vi "WPI_GyroRomiGetAngle.vi"(8 "error in":T1, 11 "GyroDevRef":typedef) -> (0 "error out":T1, 1 "Anglular Rate":T2, 2 "Angle":T2, 3 "GyroDevRef":typedef, 4 "Calibrated?":boolean)   [LabVIEW 2019]
doc: "Returns the angle, in degrees from the original heading, that the robot is currently facing.\n\nThis software is licensed. Open the labview\\readme\\WPI Robotics Library Open Source License.txt file for more information."
uses:
  <vilib>/Rock Robotics/WPI/Gyro/WPI_GyroDevRef.ctl
  <vilib>/Rock Robotics/SystemInterfaces/AI/FPGA_AIChannel.ctl
  <vilib>/Rock Robotics/SystemInterfaces/spilib/spi_bus.ctl
  <vilib>/Rock Robotics/SystemInterfaces/System/FPGA_SystemGet.vi
  <vilib>/Rock Robotics/SystemInterfaces/System/FPGA_SystemStart Async Agent.vi
  <vilib>/Rock Robotics/SystemInterfaces/System/FPGA_SystemFPGA Ref Global.vi
  <vilib>/Rock Robotics/SystemInterfaces/AI/FPGA_ReadAI.vi
  <vilib>/Rock Robotics/WPI/Simulation/Protocol/Devices/Gyro/Gyro Update Ops.ctl
panel:
  # "Analog"
  # "XRS"
  # "Analog"
  # "XRS"
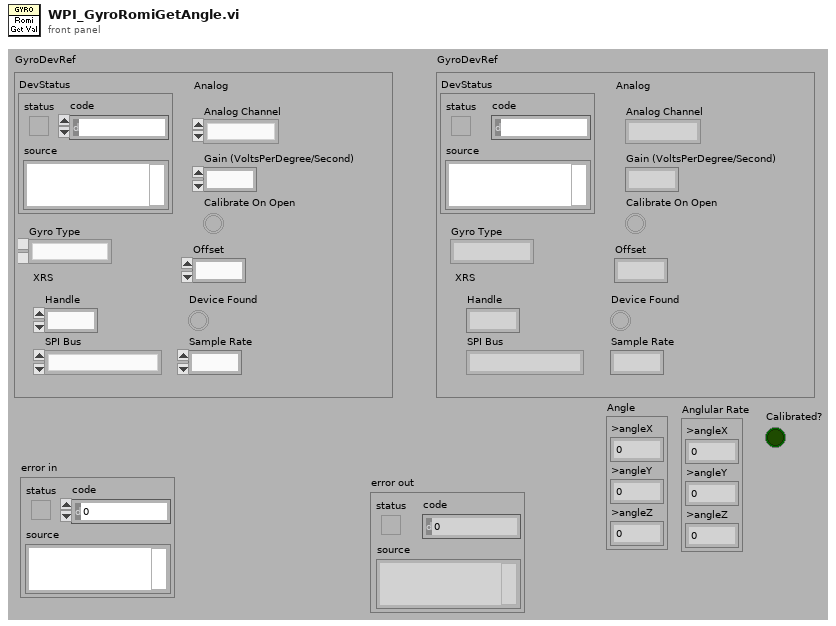
[diagram p1: front panel]
types:
  T1 = cluster{"source":string, "code":numeric, "status":boolean}
  T2 = cluster{">angleX":numeric, ">angleY":numeric, ">angleZ":numeric}
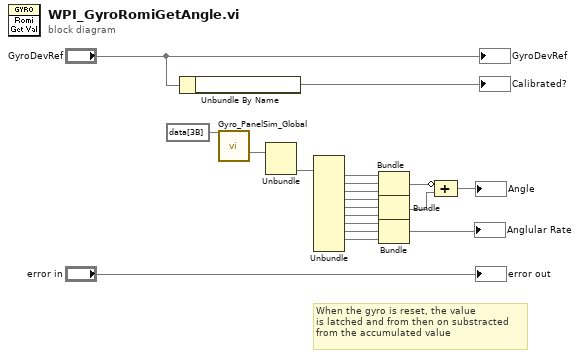
[diagram p0: block diagram]
diagram:
  w17 = data[3B] items=["get", "delete", "JSON update", "set  name", "transmit initial", "reset", "set init", "set offsetX", "set offsetY", "set offsetZ", "set gain"] ("Menu")
  # "When the gyro is reset, the value\nis latched and from then on substracted\nfrom the accumulated value"
  n1 = Unbundle By Name("GyroDevRef") -> (→"Calibrated?")
  n2 = call <vilib>:"Gyro_PanelSim_Global.vi"(0:w17) -> (10:w16)  [unwired: 13 in, 1 out]
  n3 = Unbundle(w16) -> (w15)  [unwired: 3 out]
  n4 = Unbundle(w15) -> (w4, w5, w6, w14, w13, w12, w11, w10, w9)  [unwired: 3 out]
  n5 = Bundle(w4, w5, w6) -> (w3)  [unwired: 1 in]
  n6 = Bundle(w14, w13, w12) -> (w2)  [unwired: 1 in]
  n7 = Bundle(w11, w10, w9) -> (→"Anglular Rate")  [unwired: 1 in]
  n8 = Compound Arithmetic op=ADD(invert w3, w2) -> (→"Angle")
  "GyroDevRef" <- "GyroDevRef"
  "error out" <- "error in"
